vi "CommitParametersToCameraDevice.vi"(8 "error in":errorcluster, 11 "camera handle in":u64) -> (0 "error out":errorcluster, 3 "camera handle out":u64)   [LabVIEW 2019, in "PICam.lvlib"]
doc: "PicamAdvanced_CommitParametersToCameraDevice() attempts to configure a camera\ndevice with the set of parameter values stored in model (camera handle)."
uses:
  PICam.lvlib
  Picam64.dll   
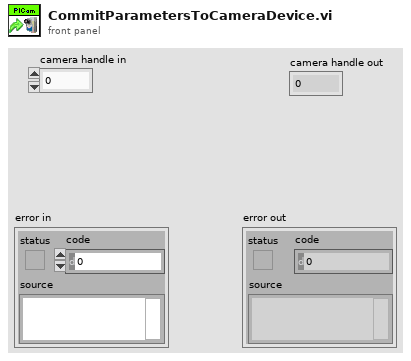
[diagram p1: front panel]
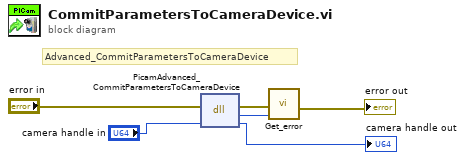
[diagram p0: block diagram]
diagram:
  # "Advanced_CommitParametersToCameraDevice"
  n1 = dll-call lib="Picam32.dll" fn="PicamAdvanced_CommitParametersToCameraDevice"(error in="error in", "camera_handle"="camera handle in") -> (error out=w5:errorcluster, "return type"=w4:i32, "camera_handle"=→"camera handle out":u64)  [unwired: 2 in, 1 out]
  n2 = call "Get_error.vi"("PICam_Error"=w4, "error in (no error)"=w5) -> ("error out"=→"error out":errorcluster)  [unwired: 9 in]
